vi "Parse Audio Item.vi"(8 "error in (no error)":errorcluster, 10 "Response":string, 11 "XBMC Ref in":T1) -> (0 "error out":errorcluster, 2 "XBMC Ref out":T1, 3 "output cluster":T3)   [LabVIEW 2013]
uses:
  Type Defs/Audio Item.ctl
  Type Defs/XBMC Ref.ctl
  <vilib>/httpClient/ClientHandle.ctl
  LMH-Kodi.lvlib
  <vilib>/httpClient/LabVIEWHTTPClient.lvlib
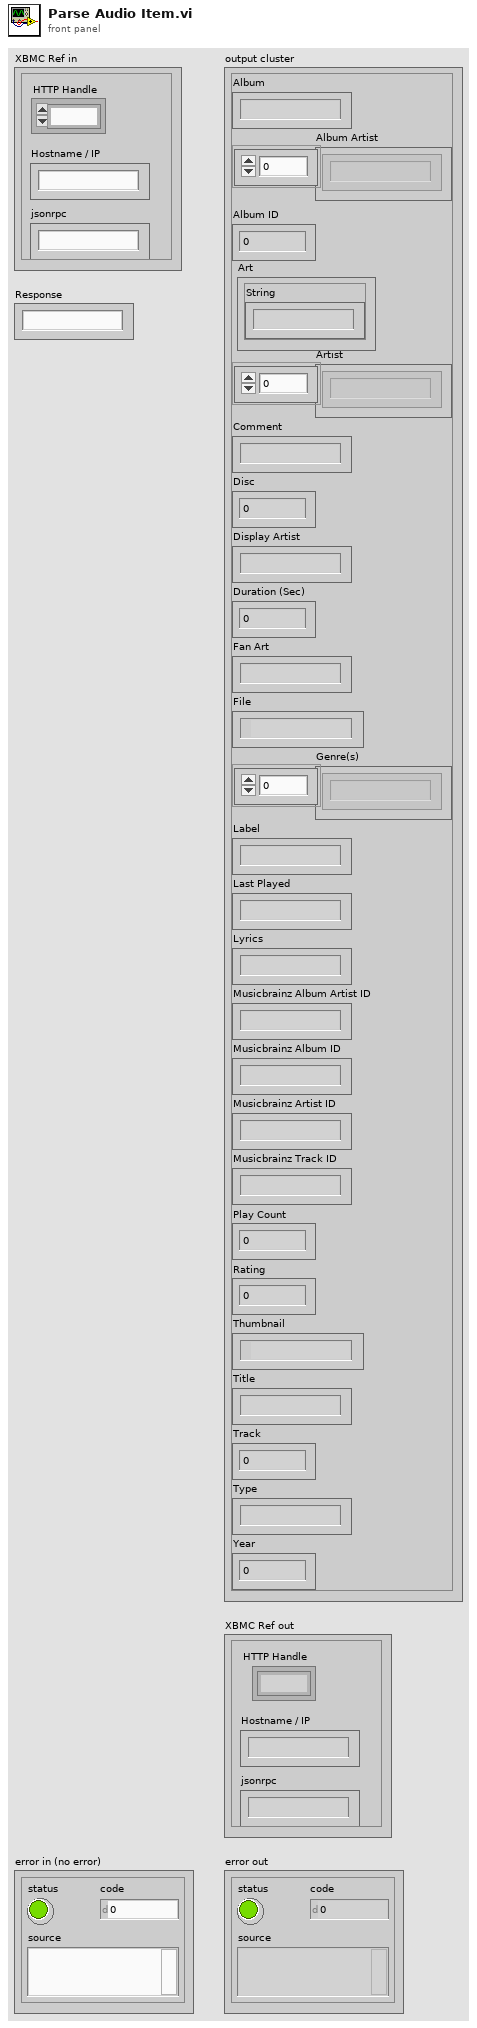
[diagram p1: front panel]
types:
  T1 = typedef "LMH-Kodi.lvlib/XBMC Ref.ctl" = cluster{"HTTP Handle":T2, "Hostname / IP":string, "jsonrpc":string}
  T2 = typedef "LabVIEWHTTPClient.lvlib/ClientHandle.ctl" = refnum<k1>
  T3 = typedef "LMH-Kodi.lvlib/Audio Item.ctl" = cluster{"Album":string, "Album Artist":string[], "Album ID":i32, "Art":cluster{"String":string}, "Artist":string[], "Comment":string, "Disc":i32, "Display Artist":string, "Duration (Sec)":i32, "Fan Art":string, "File":path, "Genre(s)":string[], "Label":string, "Last Played":string, "Lyrics":string, "Musicbrainz Album Artist ID":string, "Musicbrainz Album ID":string, "Musicbrainz Artist ID":string, "Musicbrainz Track ID":string, "Play Count":i32, "Rating":i32, "Thumbnail":path, "Title":string, "Track":i32, "Type":string, "Year":i32}
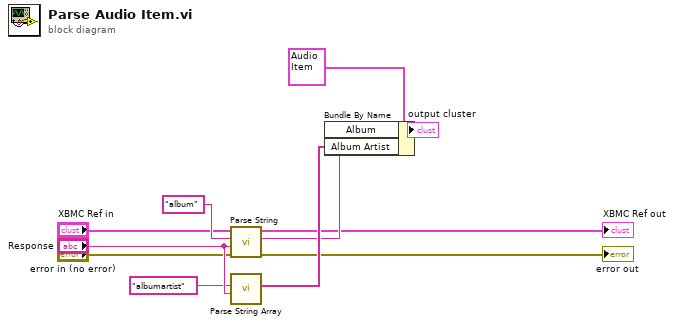
[diagram p0: block diagram]
diagram:
  n1 = call "Parse String.vi"("Error In"="error in (no error)", "JSON Response"="Response", "Key"="album", "XBMC Ref"="XBMC Ref in") -> ("Error Out"=→"error out":errorcluster, "Value"=w5:string, "XBMC Ref"=→"XBMC Ref out":T1)  [unwired: 4 in, 1 out]
  n2 = call "Parse String Array.vi"("JSON Response"="Response", "Key"="albumartist") -> ("Value"=w11:string[])  [unwired: 6 in, 3 out]
  n3 = Bundle By Name(cluster=T3 {"Album"="", "Album Artist"=[], "Album ID"=0, "Art"={"String"=""}, "Artist"=[], "Comment"="", "Disc"=0, "Display Artist"="", "Duration (Sec)"=0, "Fan Art"="", "File"=path "", "Genre(s)"=[], "Label"="", "Last Played"="", "Lyrics"="", "Musicbrainz Album Artist ID"="", "Musicbrainz Album ID"="", "Musicbrainz Artist ID"="", "Musicbrainz Track ID"="", "Play Count"=0, "Rating"=0, "Thumbnail"=path "", "Title"="", "Track"=0, "Type"="", "Year"=0} ("Audio Item"), "Album"=w5, "Album Artist"=w11) -> (→"output cluster":T3)
